vi "ma_sml_M-1 Decimator with IC (complex input).vi"(0 "x":cdb[](array[numeric]) format="%.2f", 1 "coefficients":dbl[](array[numeric]) format="%.2f", 2 "M":i32=1, 3 "initial conditions":cdb[](array[numeric]) format="%.2f", 4 "reset?":bool) -> (5 "y":cdb[](array[numeric]) format="%.2f", 6 "final conditions":cdb[](array[numeric]) format="%.2f")   [LabVIEW 2020, in "NI_MAPro.lvlib"]
doc: "Clockwise commutator implementation of polyphase M-1 decimator.\ncoefficients and initial conditions are in polyphase forms for the reason of computation efficiency.\nSince it is clockwise commutator model, output is one sample delayed at the output sample rate. the coefficients arrays are in the reverse order of ordinary polyphase filters."
uses:
  NI_MAPro.lvlib
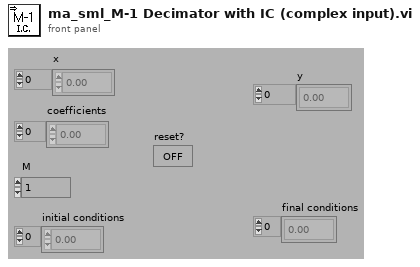
[diagram p1: front panel]
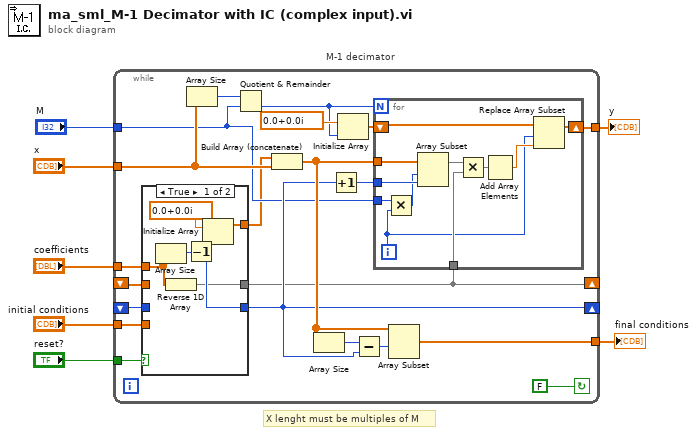
[diagram p0: block diagram]
diagram:
  # "X lenght must be multiples of M"
  # "M-1 decimator"
  n1 = while {
    tunnel: "M" -> [w11]
    tunnel: [w14] -> w2
    tunnel: [w18] -> w3
    tunnel: "coefficients" -> [w24]
    shift-left: _ -> [w23]
    shift-right: [w13] -> _
    shift-left: _ -> [w22]
    shift-right: [w10] -> _
    tunnel: "x" -> [w25]
    tunnel: "reset?" -> [w27]
    tunnel: "initial conditions" -> [w28]
    stop <- FALSE continue-if-true
    n2 = case shown="True" w27 {
      tunnel: w28 -> [_ w47]
      tunnel: [w40 w47] -> w9
      tunnel: w24 -> [w42 _]
      tunnel: [w43 w48] -> w13
      tunnel: w23 -> [_ w48]
      tunnel: [w41 w46] -> w10
      tunnel: w22 -> [_ w46]
      frame True {
        n3 = Array Size(array=w42) -> (size(s)=w44:i32)
        n4 = Reverse 1D Array(array=w42) -> (reversed array=w41:dbl[])
        n5 = Decrement(x=w44) -> (x-1=w43:i32)
        n6 = Initialize Array(cdb 0.0+0.0i ("Element Data"), w43) -> (w40:cdb[])
      }
      frame False {
      }
    }
    n7 = Array Size(array=w25) -> (size(s)=w26:i32)
    n8 = Quotient & Remainder(x=w26, y=w11) -> (floor(x/y)=w16:i32)  [unwired: 1 out]
    n9 = Build Array (concatenate)(w9, w25) -> (w21:cdb[])
    n10 = Array Size(array=w21) -> (size(s)=w20:i32)
    n11 = Increment(x=w13) -> (x+1=w12:i32)
    n12 = Initialize Array(cdb 0.0+0.0i ("Element Data"), w16) -> (w15:cdb[])
    n13 = Subtract(x=w20, y=w13) -> (x-y=w19:i32)
    n14 = for {
      N: w16 -> [_]
      tunnel: w21 -> [w38]
      shift-right: [w29] -> w14
      shift-left: w15 -> [w39]
      tunnel: w12 -> [w37]
      tunnel: w11 -> [w36]
      tunnel: w10 -> [w33]
      i -> [w30]
      n15 = Multiply(x=w36, y=w30) -> (x*y=w35:i32)
      n16 = Array Subset(array=w38, index=w35, length=w37) -> (w34:cdb[])
      n17 = Multiply(x=w34, y=w33) -> (x*y=w32:cdb[])
      n18 = Add Array Elements(numeric array=w32) -> (sum=w31:cdb)
      n19 = Replace Array Subset(array=w39, new element=w31, index=w30) -> (w29:cdb[])
    }
    n20 = Array Subset(array=w21, index=w19) -> (w18:cdb[])  [unwired: 1 in]
  }
  "y" <- w2
  "final conditions" <- w3
